vi "_Search Top Variable Source File in Map.vi"(7 "String (section)":string, 8 "error in (no error)":errorcluster, 10 "Content (key)":string, 11 "Variable-FileMap":variant) -> (0 "error out":errorcluster, 2 "Top File Path":path, 3 "Variant":variant)   [LabVIEW 2017, in "INI-Static-Variable-Support.lvlib" / "CSM-Static-Variable-Manager.lvclass"]
uses:
  CSM-Static-Variable-Manager.lvclass
  <userlib>/_NEVSTOP/Communicable State Machine(CSM)/addons/API-String-Arugments-Support/API String Arguments Support.lvlib
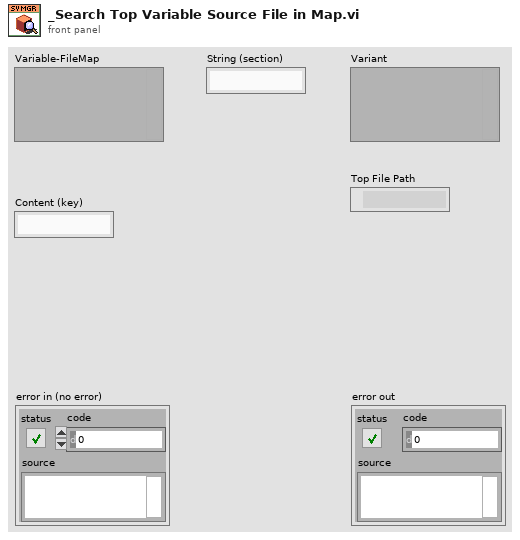
[diagram p1: front panel]
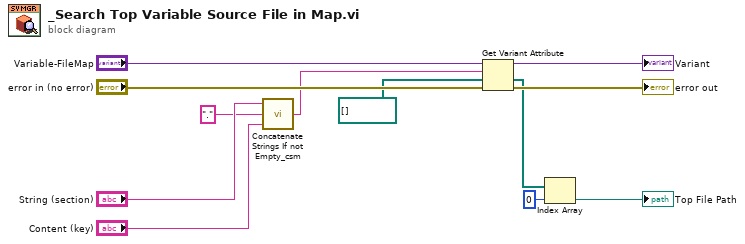
[diagram p0: block diagram]
diagram:
  n1 = call <userlib>:"Concatenate Strings If not Empty_csm.vi"("String"="Content (key)", "seperator(:)"=".", "prefix"="String (section)") -> ("result"=w9:string)  [unwired: 2 in]
  n2 = Get Variant Attribute(Variant="Variable-FileMap", name=w9, default value (empty Variant)=path[] [], error in="error in (no error)") -> (duplicate Variant=→"Variant":variant, value=w1:path[], error out=→"error out":errorcluster)  [unwired: 1 out]
  n3 = Index Array(array=w1, index=0) -> (element=→"Top File Path":path)
